vi "Build EthernetFrame (IP).vi"(7 "Calculate Checksum Internally?":bool=TRUE, 10 "IP header":T1 {"Dest IP" format="%x"; "Source IP" format="%x"; "Checksum" format="%x"; "Protocol" format="%x"; "TTL" format="%x"; "FragOffset" format="%x"; "ID" format="%x"; "Lenght" format="%x"; "QoS" format="%x"; "IHL" format="%x"; "Version" format="%x"}, 11 "Ethernet Frame In":u8[](array[numeric]) format="%.0x") -> (3 "Ethernet Frame Out":u8[](array[numeric]) format="%.0x")   [LabVIEW 2020, in "EthFrameManagement.lvlib"]
doc: "Build an Ethernet frame based in the IP header."
uses:
  EthFrameManagement.lvlib
  controls/IPFrame_type.ctl
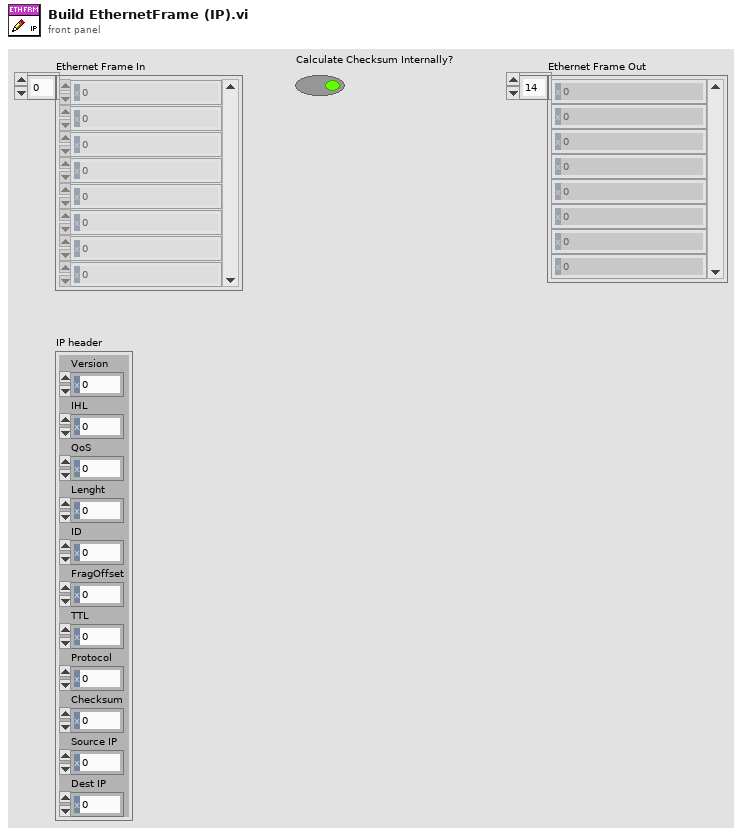
[diagram p1: front panel]
types:
  T1 = typedef "EthFrameManagement.lvlib/IPFrame_type.ctl" = cluster{"Version":u8, "IHL":u8, "QoS":u8, "Lenght":u16, "ID":u16, "FragOffset":u16, "TTL":u8, "Protocol":u8, "Checksum":u16, "Source IP":u32, "Dest IP":u32}
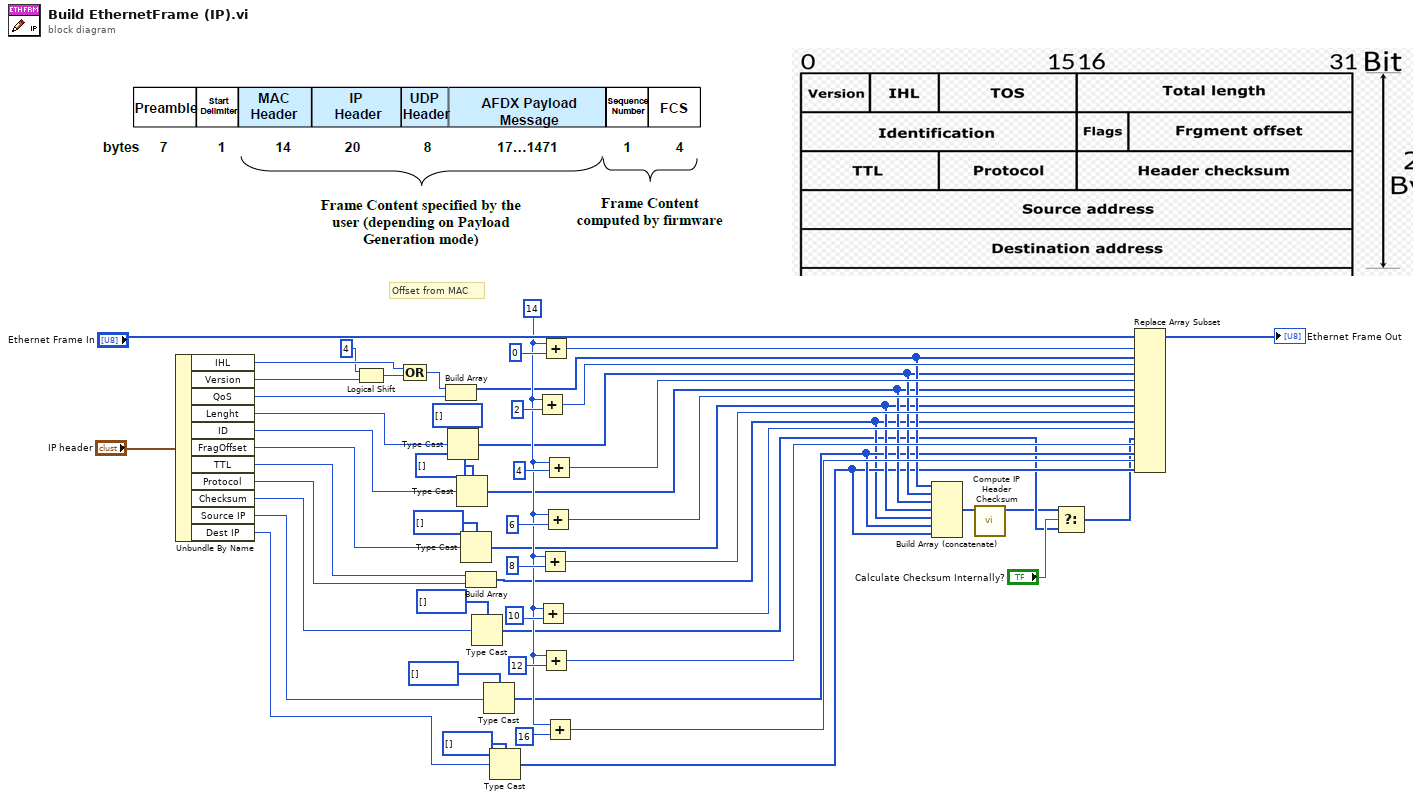
[diagram p0: block diagram]
diagram:
  w15 = 14 ("length")
  # "Offset from MAC"
  n1 = Unbundle By Name("IP header") -> ("IHL"=w47:u8, "Version"=w49:u8, "QoS"=w40:u8, "Lenght"=w39:u16, "ID"=w32:u16, "FragOffset"=w29:u16, "TTL"=w27:u8, "Protocol"=w26:u8, "Checksum"=w24:u16, "Source IP"=w43:u32, "Dest IP"=w42:u32)
  n2 = Logical Shift(y=i16 4, x=w49) -> (x << y=w48:u8)
  n3 = Compound Arithmetic op=OR(w47, w48) -> (w45:u8)
  n4 = Build Array(w45, w40) -> (w12:u8[])
  n5 = Type Cast(type=u8[] [] ("Ethernet Frame In"), x=w39) -> (*(type *) &x=w11:u8[])
  n6 = Type Cast(type=u8[] [] ("Ethernet Frame In"), x=w32) -> (*(type *) &x=w10:u8[])
  n7 = Type Cast(type=u8[] [] ("Ethernet Frame In"), x=w29) -> (*(type *) &x=w9:u8[])
  n8 = Build Array(w27, w26) -> (w4:u8[])
  n9 = Type Cast(type=u8[] [] ("Ethernet Frame In"), x=w24) -> (*(type *) &x=w3:u8[])
  n10 = Type Cast(type=u8[] [] ("Ethernet Frame In"), x=w43) -> (*(type *) &x=w8:u8[])
  n11 = Type Cast(type=u8[] [] ("Ethernet Frame In"), x=w42) -> (*(type *) &x=w7:u8[])
  n12 = Add(x=w15, y=2 ("length")) -> (x+y=w34:i32)
  n13 = Add(x=w15, y=10 ("length")) -> (x+y=w18:i32)
  n14 = Add(x=w15, y=8 ("length")) -> (x+y=w20:i32)
  n15 = Add(x=w15, y=0 ("length")) -> (x+y=w37:i32)
  n16 = Add(x=w15, y=12 ("length")) -> (x+y=w17:i32)
  n17 = Add(x=w15, y=6 ("length")) -> (x+y=w28:i32)
  n18 = Add(x=w15, y=4 ("length")) -> (x+y=w31:i32)
  n19 = Add(x=w15, y=16 ("length")) -> (x+y=w13:i32)
  n20 = Build Array (concatenate)(w12, w11, w10, w9, w4, w8, w7) -> (w6:u8[])
  n21 = call "Compute IP Header Checksum.vi"("IP Header"=w6) -> ("Checksum"=w2:u8[])  [unwired: 10 in]
  n22 = Select(t=w2, s="Calculate Checksum Internally?", f=w3) -> (s? t:f=w1:u8[])
  n23 = Replace Array Subset(array="Ethernet Frame In", new element #1=w12, index #1=w37, new element #2=w11, index #2=w34, new element #3=w10, index #3=w31, new element #4=w9, index #4=w28, new element #5=w4, index #5=w20, new element #6=w1, index #6=w18, new element #7=w8, index #7=w17, new element #8=w7, index #8=w13) -> (→"Ethernet Frame Out":u8[])
